vi "Acquire Ring Time.vi"(8 "error in (no error)":errorcluster, 11 "Settings In":T1) -> (0 "error out":errorcluster, 3 "Settings Out":T1)   [LabVIEW 2019, in "Acquisition.lvlib"]
uses:
  <vilib>/DAQmx/read.llb/DAQmx Read (Analog 1D Wfm NChan NSamp).vi
  <vilib>/DAQmx/miscellaneous.llb/DAQmx Fill In Error Info.vi
  Acquisition.lvlib
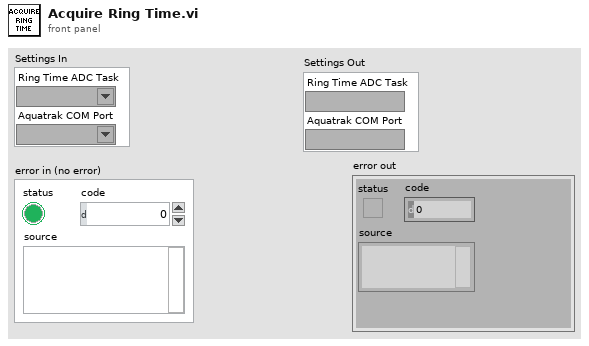
[diagram p1: front panel]
types:
  T1 = cluster{"Ring Time ADC Task":refnum<k21>, "Aquatrak COM Port":refnum<visa-resource-name>}
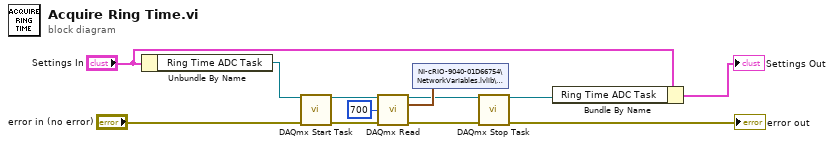
[diagram p0: block diagram]
diagram:
  n1 = Unbundle By Name("Settings In") -> ("Ring Time ADC Task"=w11:refnum<k21>)
  n2 = call <vilib>:"DAQmx Start Task.vi"("task/channels in"=w11, "error in"="error in (no error)") -> ("task out"=w8:refnum<k21>, "error out"=w5:errorcluster)  [unwired: 12 in]
  n3 = call-poly <vilib>:"DAQmx Read.vi"("task/channels in"=w8, "number of samples per channel"=700, "error in"=w5) -> ("task out"=w7:refnum<k21>, "data"=w10:waveform(dbl)[], "error out"=w6:errorcluster)  [unwired: 10 in]
  n4 = shared-variable "NI-cRIO-9040-01D66754\\NetworkVariables.lvlib\\RingTime"(w10) -> ()  [unwired: 1 in, 1 out]
  n5 = call <vilib>:"DAQmx Stop Task.vi"("task/channels in"=w7, "error in"=w6) -> ("task out"=w1:refnum<k21>, "error out"=→"error out":errorcluster)  [unwired: 12 in]
  n6 = Bundle By Name(cluster="Settings In", "Ring Time ADC Task"=w1) -> (→"Settings Out":T1)
